vi "Configure Basic Digitizer.vi"(6 "Jitter Detection (0: AllBits)":i32(ring) items=["AllBits", "StableBits", "Preamble", "SqRising", "SqFalling", "SqBoth"], 7 "Input Gain (0: dgAuto)":i32(ring) items=["dgAuto", "dgx1", "dgx2", "dgx4"], 8 "error in (no error)":errorcluster, 9 "Repeat Acquistion (T: Enable)":bool=TRUE, 10 "Record Length (0: drl4k)":i32(ring) items=["drl4k", "drl8k", "drl16k", "drl32k", "drl64k", "drl128k", "drl256k", "drl512k", "drl1M", "drl2M"], 11 "VISA resource name":refnum<visa-resource-name>) -> (0 "error out":errorcluster, 3 "VISA resource name out":refnum<visa-resource-name>)   [LabVIEW 2014, in "Stanford Research SR1.lvlib"]
doc: "Configures the basic attributes of the Digitzer."
uses:
  Stanford Research SR1.lvlib
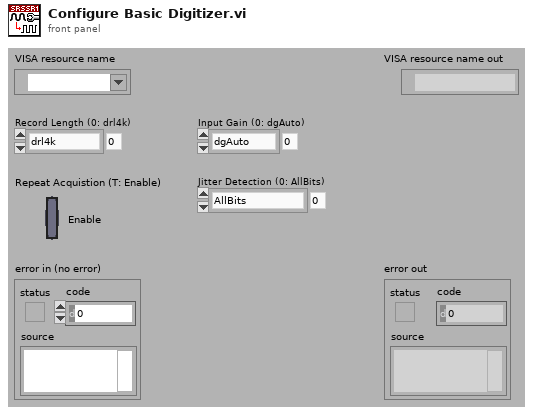
[diagram p1: front panel]
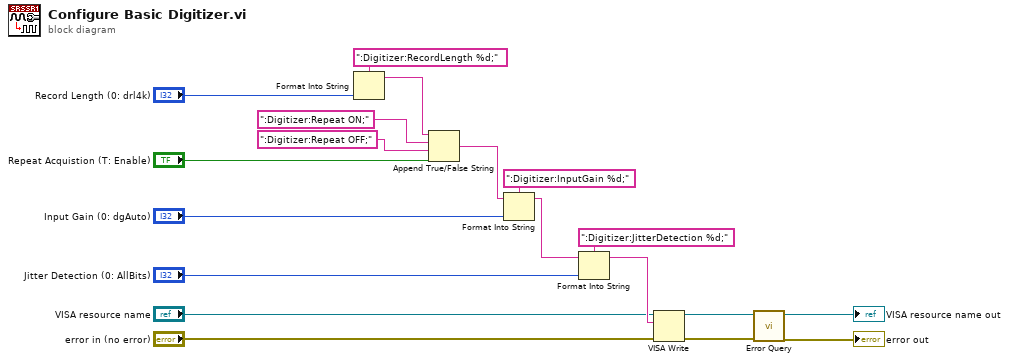
[diagram p0: block diagram]
diagram:
  n1 = Format Into String(format string=":Digitizer:RecordLength %d;", "Record Length (0: drl4k)") -> (resulting string=w17:string)  [unwired: 2 in, 1 out]
  n2 = Append True/False String(1:"Repeat Acquistion (T: Enable)", 2:":Digitizer:Repeat OFF;", 3:":Digitizer:Repeat ON;", 4:w17) -> (0:w13:string)
  n3 = Format Into String(format string=":Digitizer:InputGain %d;", initial string=w13, "Input Gain (0: dgAuto)") -> (resulting string=w10:string)  [unwired: 1 in, 1 out]
  n4 = Format Into String(format string=":Digitizer:JitterDetection %d;", initial string=w10, "Jitter Detection (0: AllBits)") -> (resulting string=w7:string)  [unwired: 1 in, 1 out]
  n5 = VISA Write(VISA resource name="VISA resource name", write buffer=w7, error in (no error)="error in (no error)") -> (VISA resource name out=w4:refnum<visa-resource-name>, error out=w3:errorcluster)  [unwired: 1 out]
  n6 = call "Error Query.vi"("error in (no error)"=w3, "VISA resource name"=w4) -> ("error out"=→"error out":errorcluster, "VISA resource name out"=→"VISA resource name out":refnum<visa-resource-name>)  [unwired: 6 in, 2 out]
